vi "Finish.vi"(8 "error in (no error)":errorcluster, 11 "Hatch Concrete in":refnum<class "Hatch Concrete.lvclass">) -> (0 "error out":errorcluster, 3 "Hatch Concrete out":refnum<class "Hatch Concrete.lvclass">)   [LabVIEW 2019, in "Hatch.lvlib" / "Hatch Concrete.lvclass"]
doc: "Closes referances for the hatch."
uses:
  Hatch Concrete.lvclass
  Hatch.lvclass
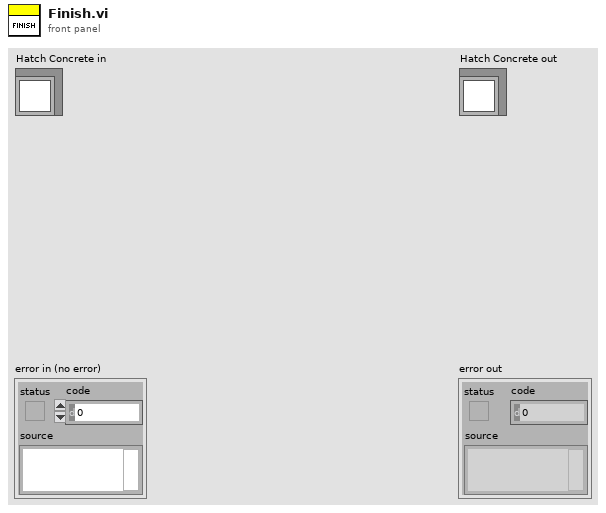
[diagram p1: front panel]
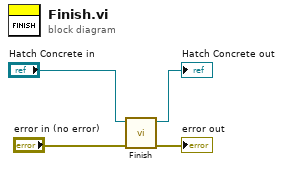
[diagram p0: block diagram]
diagram:
  n1 = call-parent "Finish.vi"("error in (no error)"="error in (no error)", "Hatch in"="Hatch Concrete in") -> ("error out"=→"error out":errorcluster, "Hatch out"=→"Hatch Concrete out":refnum<class "Hatch Concrete.lvclass">)  [unwired: 8 in]
